vi "pumpStatus.vi"(0 "VISA resource name":refnum<visa-resource-name>, 11 "error in (no error)":errorcluster) -> (4 "PumpKW":dbl, 6 "PumpTemp":u16, 8 "PumpAmps":dbl, 10 "PumpVolts":dbl, 14 "TurboSpeed":dbl(knob) scale=0.0..100.0, 15 "error out":errorcluster)   [LabVIEW 2013]
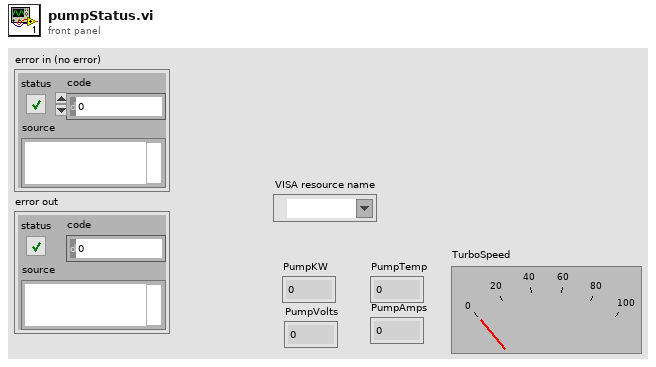
[diagram p1: front panel]
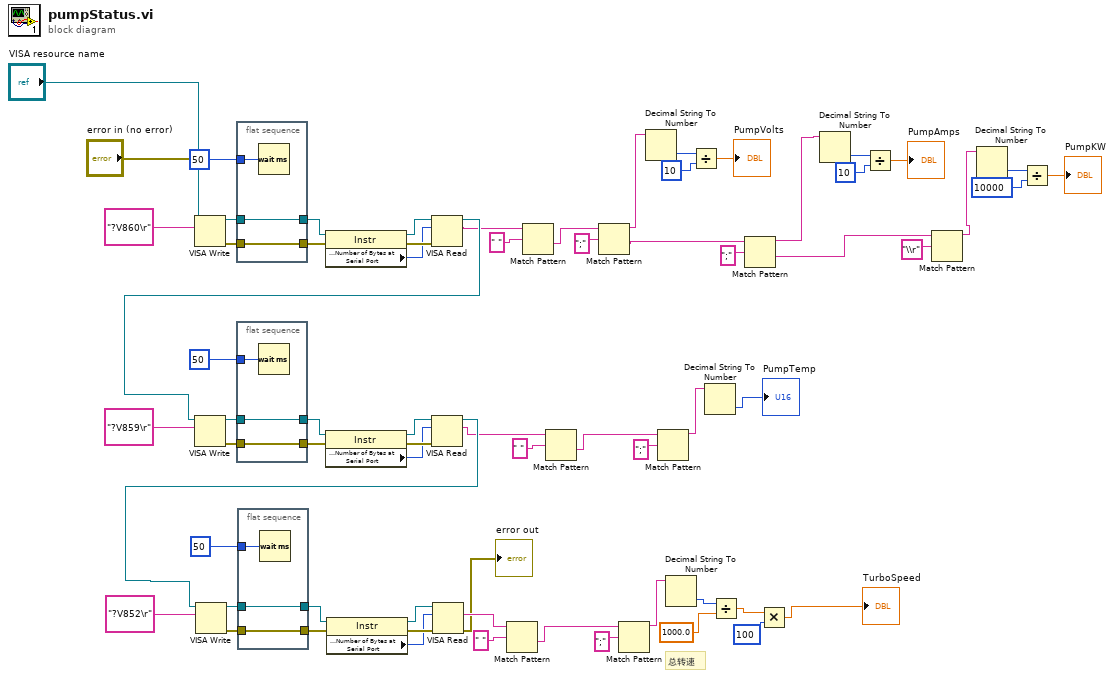
[diagram p0: block diagram]
diagram:
  # "总转速"
  n1 = VISA Write(VISA resource name="VISA resource name", write buffer="?V860\r" ("Command"), error in (no error)="error in (no error)") -> (VISA resource name out=w13:refnum<visa-resource-name>, error out=w15:errorcluster)  [unwired: 1 out]
  n2 = flat-sequence {
    tunnel: w15 -> [w70]
    tunnel: [w70] -> w14
    tunnel: w13 -> [w69]
    tunnel: [w69] -> w12
    tunnel: u32 50 ("delay before read (ms)") -> [w71]
    frame #0 {
      n3 = Wait (ms)(milliseconds to wait=w71) -> ()  [unwired: 1 out]
    }
  }
  n4 = flat-sequence {
    tunnel: w44 -> [w73]
    tunnel: [w73] -> w43
    tunnel: w42 -> [w72]
    tunnel: [w72] -> w41
    tunnel: u32 50 ("delay before read (ms)") -> [w74]
    frame #0 {
      n5 = Wait (ms)(milliseconds to wait=w74) -> ()  [unwired: 1 out]
    }
  }
  n6 = flat-sequence {
    tunnel: w60 -> [w76]
    tunnel: [w76] -> w59
    tunnel: w58 -> [w75]
    tunnel: [w75] -> w57
    tunnel: u32 50 ("delay before read (ms)") -> [w77]
    frame #0 {
      n7 = Wait (ms)(milliseconds to wait=w77) -> ()  [unwired: 1 out]
    }
  }
  n8 = property class="Instr"(reference=w12, error in=w14) -> (reference out=w10:refnum<visa-resource-name>, error out=w9:errorcluster, "Serial Settings:Number of Bytes at Serial Port"=w8:u32)
  n9 = property class="Instr"(reference=w41, error in=w43) -> (reference out=w39:refnum<visa-resource-name>, error out=w38:errorcluster, "Serial Settings:Number of Bytes at Serial Port"=w37:u32)
  n10 = property class="Instr"(reference=w57, error in=w59) -> (reference out=w55:refnum<visa-resource-name>, error out=w54:errorcluster, "Serial Settings:Number of Bytes at Serial Port"=w53:u32)
  n11 = VISA Read(VISA resource name=w10, byte count=w8, error in (no error)=w9) -> (VISA resource name out=w45:refnum<visa-resource-name>, read buffer=w25:string)  [unwired: 2 out]
  n12 = VISA Write(VISA resource name=w45, write buffer="?V859\r" ("Command")) -> (VISA resource name out=w42:refnum<visa-resource-name>, error out=w44:errorcluster)  [unwired: 1 in, 1 out]
  n13 = VISA Read(VISA resource name=w39, byte count=w37, error in (no error)=w38) -> (VISA resource name out=w61:refnum<visa-resource-name>, read buffer=w50:string)  [unwired: 2 out]
  n14 = VISA Write(VISA resource name=w61, write buffer="?V852\r" ("Command")) -> (VISA resource name out=w58:refnum<visa-resource-name>, error out=w60:errorcluster)  [unwired: 1 in, 1 out]
  n15 = VISA Read(VISA resource name=w55, byte count=w53, error in (no error)=w54) -> (read buffer=w66:string, error out=→"error out":errorcluster)  [unwired: 2 out]
  n16 = Match Pattern(string=w66, regular expression=" ") -> (after substring=w63:string)  [unwired: 1 in, 3 out]
  n17 = Match Pattern(string=w25, regular expression=" ") -> (after substring=w27:string)  [unwired: 1 in, 3 out]
  n18 = Match Pattern(string=w50, regular expression=" ") -> (after substring=w47:string)  [unwired: 1 in, 3 out]
  n19 = Match Pattern(string=w27, regular expression=";") -> (before substring=w29:string, after substring=w31:string)  [unwired: 1 in, 2 out]
  n20 = Match Pattern(string=w63, regular expression=";") -> (before substring=w65:string)  [unwired: 1 in, 3 out]
  n21 = Decimal String To Number(string=w29) -> (number=w16:i32)  [unwired: 2 in, 1 out]
  n22 = Match Pattern(string=w47, regular expression=";") -> (before substring=w49:string)  [unwired: 1 in, 3 out]
  n23 = Decimal String To Number(string=w65) -> (number=w67:i32)  [unwired: 2 in, 1 out]
  n24 = Divide(x=w16, y=10) -> (x/y=→"PumpVolts":dbl)
  n25 = Decimal String To Number(string=w49) -> (number=→"PumpTemp":i32)  [unwired: 2 in, 1 out]
  n26 = Divide(x=w67, y=1000.0) -> (x/y=w3:dbl)
  n27 = Match Pattern(string=w31, regular expression=";") -> (before substring=w32:string, after substring=w34:string)  [unwired: 1 in, 2 out]
  n28 = Multiply(x=w3, y=100) -> (x*y=→"TurboSpeed":dbl)
  n29 = Decimal String To Number(string=w32) -> (number=w19:i32)  [unwired: 2 in, 1 out]
  n30 = Divide(x=w19, y=10) -> (x/y=→"PumpAmps":dbl)
  n31 = Match Pattern(string=w34, regular expression="\\r") -> (before substring=w35:string)  [unwired: 1 in, 3 out]
  n32 = Decimal String To Number(string=w35) -> (number=w22:i32)  [unwired: 2 in, 1 out]
  n33 = Divide(x=w22, y=10000) -> (x/y=→"PumpKW":dbl)
